vi "sendMessage.vi"(8 "error in (no error)":errorcluster, 9 "data":variant, 10 "message":string, 11 "MsgUETaskChannel in":refnum<class "MsgUETaskChannel.lvclass">) -> (0 "error out":errorcluster, 3 "MsgUETaskChannel out":refnum<class "MsgUETaskChannel.lvclass">)   [LabVIEW 2023, in "TLC_Daemon.lvlib" / "MsgUETaskChannel.lvclass"]
uses:
  MsgUETaskChannel.lvclass
  Ctrls/msg.ctl
  MsgUETaskChannel.lvclass/MsgUETaskChannel.ctl
  TLC_Daemon.lvlib
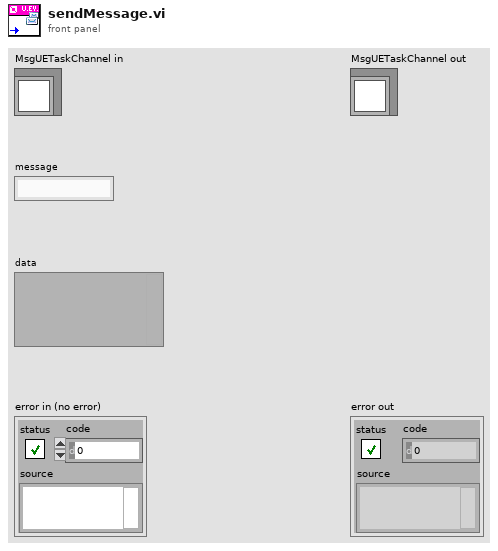
[diagram p1: front panel]
types:
  T1 = typedef "TLC_Daemon.lvlib/msg.ctl" = cluster{"message":string, "data":variant}
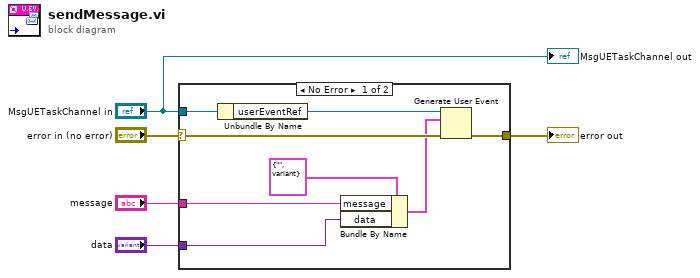
[diagram p0: block diagram]
diagram:
  n1 = case shown="No Error" "error in (no error)" {
    selector: "error in (no error)" -> [w10 w14]
    tunnel: [w11 w14] -> w4
    tunnel: "MsgUETaskChannel in" -> [w13 _]
    tunnel: "message" -> [w8 _]
    tunnel: "data" -> [w7 _]
    frame No Error {
      n2 = Unbundle By Name(w13) -> ("userEventRef"=w12:refnum<user-event>)
      n3 = Bundle By Name(cluster=T1 {"message"="", "data"=variant} ("event data"), "message"=w8, "data"=w7) -> (w6:T1)
      n4 = Generate User Event(user event=w12, event data cluster=w6, error in=w10) -> (error out=w11:errorcluster)  [unwired: 1 in, 1 out]
    }
    frame Error {
    }
  }
  "error out" <- w4
  "MsgUETaskChannel out" <- "MsgUETaskChannel in"
